vi "Reformat Cal Inst data files.vi"(11 "file path (dialog if empty)":path=path "C:/Users/dhstuart/Dropbox/CLTC/LED life testing/temp1.WFD") -> (3 "Electrical Data":T1)   [LabVIEW 2013]
uses:
  electrical.ctl
  <vilib>/Utility/file.llb/Read From Spreadsheet File (string).vi
panel:
  out "Electrical data labels":string[](array[string])
  out "Electrical data":string[](array[string])
  out "Current Waverform":waveform(dbl)(graph)
  out "Voltage Waveform":waveform(dbl)(graph)
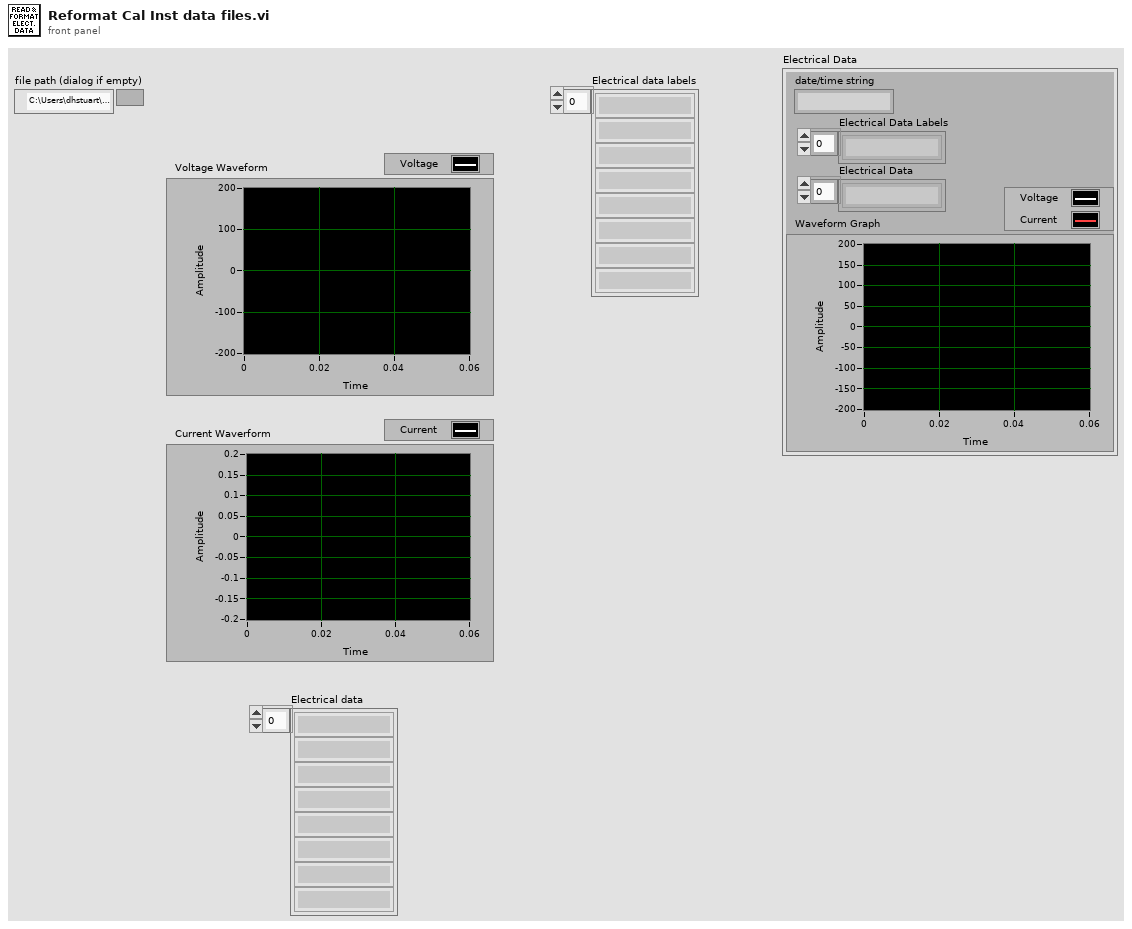
[diagram p1: front panel]
types:
  T1 = typedef "electrical.ctl" = cluster{"date/time string":string, "Electrical Data Labels":string[], "Electrical Data":string[], "Waveform Graph":waveform(dbl)[]}
  T2 = cluster{"date/time string":string, string[], string[], waveform(dbl)[]}
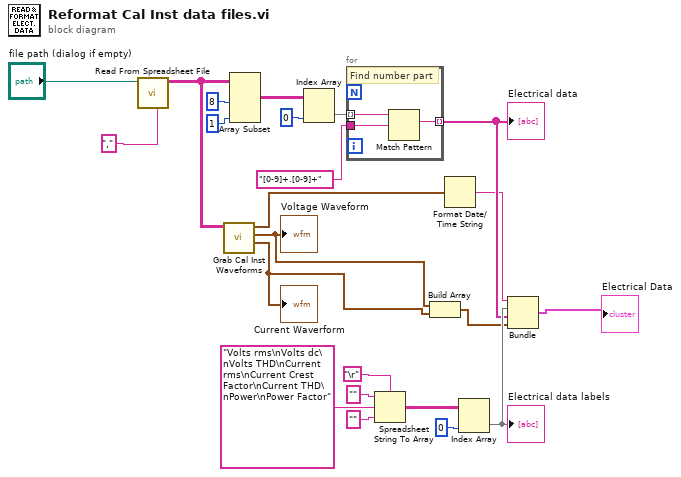
[diagram p0: block diagram]
diagram:
  n1 = call-poly <vilib>:"Read From Spreadsheet File.vi"("delimiter (\\t)"="," ("delimiter (\\t)"), "file path (dialog if empty)"="file path (dialog if empty)") -> ("all rows"=w7:string[][])  [unwired: 5 in, 4 out]
  n2 = call "Grab Cal Inst Waveforms.vi"("all rows"=w7) -> ("Current Waverform"=w3:waveform(dbl), "Voltage Waveform"=w4:waveform(dbl), "Resulting Time Stamp"=w6:timestamp)  [unwired: 8 in]
  "Voltage Waveform" <- w4
  "Current Waverform" <- w3
  n3 = Array Subset(array=w7, length (row)=8 ("length"), length (col)=1 ("length")) -> (w18:string[][])  [unwired: 2 in]
  n4 = Index Array(array=w18, index (col)=0 ("disabled index (col)")) -> (element=w17:string[])  [unwired: 1 in]
  n5 = for {
    tunnel: w17 -> [w26] mode=indexing
    tunnel: [w25] -> w8 mode=indexing
    tunnel: "[0-9]+.[0-9]+" ("regular expression") -> [w24]
    # "Find number part"
    n6 = Match Pattern(string=w26, regular expression=w24) -> (match substring=w25:string)  [unwired: 1 in, 3 out]
  }
  "Electrical data" <- w8
  n7 = Spreadsheet String To Array(delimiter (Tab)="\r", format string="", spreadsheet string="Volts rms\nVolts dc\nVolts THD\nCurrent rms\nCurrent Crest Factor\nCurrent THD\nPower\nPower Factor", array type (2D Dbl)="") -> (array=w10:string[][])
  n8 = Build Array(w4, w3) -> (w2:waveform(dbl)[])
  n9 = Format Date/Time String(seconds (now)=w6) -> (date/time string=w5:string)  [unwired: 2 in]
  n10 = Index Array(array=w10, index (col)=0) -> (element=w9:string[])  [unwired: 1 in]
  "Electrical data labels" <- w9
  n11 = Bundle("date/time string"=w5, w9, w8, w2) -> (→"Electrical Data":T2)  [unwired: 1 in]
